vi "Teleop.vi"(10 "Match Info":T1={"Autonomous Elapsed Seconds"=0.0, "TeleOp Elapsed Seconds"=0.0, "Disabled Elapsed Seconds"=0.0, "Visited Autonomous"=FALSE, "Visited TeleOp"=FALSE, "Visited Disabled"=FALSE, "Autonomous Settings"={"Autonomous Style"=enum."Independent", "VI Refnum"=refnum}}, 11 "Call Context":T2) -> ()   [LabVIEW 2015]
doc: "This VI is called for each TeleOp packet received from the DS where the robot is not disabled. It is often used to read from the joysticks and update I/O or to update setpoints for timed control loops. It should complete and return within 20 milliseconds or it may miss DS packets."
uses:
  <vilib>/Rock Robotics/WPI/DriverStation/WPI_DriverStationDerivedRobotMode.ctl
  <vilib>/Rock Robotics/WPI/DriverStation/WPI_DriverStationMatch Info.ctl
  <vilib>/Rock Robotics/WPI/Utilities/WPI_GetSetVariantRefNum.vi
  <vilib>/Rock Robotics/Network Tables/SD Write Number.vi
  Robot Global Data.vi
  <vilib>/Rock Robotics/WPI/Solenoid/Deprecated/WPI_SolenoidSetBool.vi
  Z navX/navX Library v2/navX Library v2.lvlib
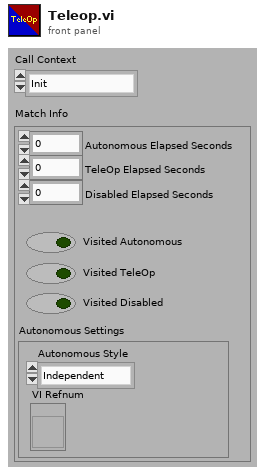
[diagram p1: front panel]
types:
  T1 = typedef "WPI_DriverStationMatch Info.ctl" = cluster{"Autonomous Elapsed Seconds":dbl, "TeleOp Elapsed Seconds":dbl, "Disabled Elapsed Seconds":dbl, "Visited Autonomous":bool, "Visited TeleOp":bool, "Visited Disabled":bool, "Autonomous Settings":cluster{"Autonomous Style":enum16{"Iterative", "Independent"}, "VI Refnum":refnum<vi>}}
  T2 = typedef "WPI_DriverStationDerivedRobotMode.ctl" = enum16{"Init", "Execute", "Stop"}
  T3 = enum16{"No Override", "Override to Coast", "Override to Brake"}
  T4 = typedef "WPI_JoystickDevRef.ctl" = cluster{"Device":T5}
  T5 = typedef "WPI_JoystickDeviceEnum.ctl" = enum16{"USB 0", "USB 1", "USB 2", "USB 3", "USB 4", "USB 5"}
  T6 = cluster{"Axes[0]":dbl, "Axes[1]":dbl, "Axes[2]":dbl, "Axes[3]":dbl, "Axes[4]":dbl, "Axes[5]":dbl, "Axes[6]":dbl, "Axes[7]":dbl, "Axes[8]":dbl}
  T7 = cluster{"Buttons[0]":bool, "Buttons[1]":bool, "Buttons[2]":bool, "Buttons[3]":bool, "Buttons[4]":bool, "Buttons[5]":bool, "Buttons[6]":bool, "Buttons[7]":bool, "Buttons[8]":bool}
  T8 = typedef "navX Library v2.lvlib/Z900_navX_DeviceTypeDef.ctl" = cluster{"Interface":cluster{"Protocol":T9, "Update Rate (4Hz-60Hz)":u8, "navX Open TypeDef":variant}, "Notify Packet":refnum<notifier>, "Loop VI Refnum":refnum<vi>, "Ready to Close Occurrence Refnum":refnum<k4>}
  T9 = typedef "navX Library v2.lvlib/Z900_navX_ProtocolTypeDef.ctl" = enum16{"SERIAL", "I2C", "SPI"}
  T10 = cluster{"Yaw":dbl, "Roll":dbl, "Pitch":dbl, "Heading":dbl, "Fused Heading":dbl}
  T11 = cluster{"LinearAcceleration X":dbl, "LinearAcceleration Y":dbl, "LinearAcceleration Z":dbl}
  T12 = cluster{"Velocity X":dbl, "Velocity Y":dbl, "Velocity Z":dbl, "Displacement X":dbl, "Displacement Y":dbl, "Displacement Z":dbl}
  T13 = typedef "WPI_MotorControlDeviceRef.ctl" = cluster{"DeviceStatus":errorcluster, "Type":T14, "PWM":cluster{"PWM Channel":T15, "DeadBand":T16}, "CAN":cluster{"Device Number":u8, "Control Mode":T17, "Semaphore":T18, "Max Vout":dbl, "TalonSRX Control Mode":T19}, "Invert":bool}
  T14 = typedef "WPI_MotorControlType.ctl" = enum16{"PWM", "CAN", "CANTalonSRX"}
  T15 = typedef "FPGA_DIOPWMChannel.ctl" = enum8{"PWM 0", "PWM 1", "PWM 2", "PWM 3", "PWM 4", "PWM 5", "PWM 6", "PWM 7", "PWM 8", "PWM 9", "PWM MXP 0", "PWM MXP 1", "PWM MXP 2", "PWM MXP 3", "PWM MXP 4", "PWM MXP 5", "PWM MXP 6", "PWM MXP 7", "PWM MXP 8", "PWM MXP 9", "Invalid"}
  T16 = typedef "WPI_PWMDeadband.ctl" = cluster{"Name":string, "maxPositivePwm":i32, "minPositivePwm":i32, "centerPwm":i32, "maxNegativePwm":i32, "minNegativePwm":i32, "angularRange":u16}
  T17 = typedef "WPI_CANJaguar_ControlMode.ctl" = enum8{"Percent VBus", "Current", "Speed", "Position", "Voltage"}
  T18 = typedef "Semaphore RefNum" = refnum<k1>
  T19 = typedef "WPI_CANTalonSRX_APIControlMode.ctl" = enum8{"Percent VBus", "Speed", "Position", "Slave", "Unchanged / Invalid", "Voltage Compensation", "Current", "Motion Profile"}
  T20 = typedef "WPI_SolenoidDevRef.ctl" = cluster{"DevStatus":errorcluster, "Pneumatics Control Module":u8, "Forward Solenoid Channel":T21, "Reverse Solenoid Channel":T21}
  T21 = typedef "WPI_SolenoidChannel.ctl" = enum8{"Solenoid 0", "Solenoid 1", "Solenoid 2", "Solenoid 3", "Solenoid 4", "Solenoid 5", "Solenoid 6", "Solenoid 7", "Invalid"}
  T22 = typedef "WPI_CANTalonSRX_GlobalStatus.ctl" = cluster{"Applied Throttle":dbl, "Module Enabled":bool, "CAN Error":errorcluster, "Closed Loop Error":dbl, "Forward Limit Switch Closed":bool, "Reverse Limit Switch Closed":bool, "Sensor Position":dbl, "Sensor Velocity":dbl, "Current":dbl, "Sticky Fault - Over Temp":bool, "Sticky Fault - Under Voltage":bool, "Sticky Fault - Forward Limit":bool, "Sticky Fault - Reverse Limit":bool, "Sticky Fault - Forward Soft Limit":bool, "Sticky Fault - Reverse Soft Limit":bool, "Brake is Enabled":bool, "Encoder Position":dbl, "Encoder Velocity":dbl, "Encoder Index Count":dbl, "Encoder A Pin State":bool, "Encoder B Pin State":bool, "Encoder Index Pin State":bool, "Analog In":dbl, "Analog In Velocity":dbl, "Temperature (C)":dbl, "Battery Voltage":dbl, "Control 5 Is Supported":bool, "Current Profile Slot Select":dbl, "Pos Div 8":bool, "Vel Div 4":bool, "Pulse Width Position":i32, "Pulse Width Velocity":i32, "Pulse Width Rise To Rise (us)":i32, "Pulse Width Rise To Fall (us)":i32, "Mot Prof Active Is Under Run":bool, "Mot Prof Active Has Under Run":bool, "Mot Prof Active Is Last":bool, "Mot Prof Active Velocity Only":bool, "Mot Prof Active Is Valid":bool, "Mot Prof Buffer Is Full":bool, "Mot Prof Active Profile Slot Select":i32, "Mot Prof NextID":i32, "Mot Prof Count":i32, "Mot Prof Active Velocity":dbl, "Mot Prof Active Position":dbl, "Mot Prof Output Enable":i32}
  T23 = typedef "WPI_RobotDriveDevRef.ctl" = cluster{"DevStatus":errorcluster, "Motors[]":T13[], "Square Inputs":bool, "Max Output":dbl}
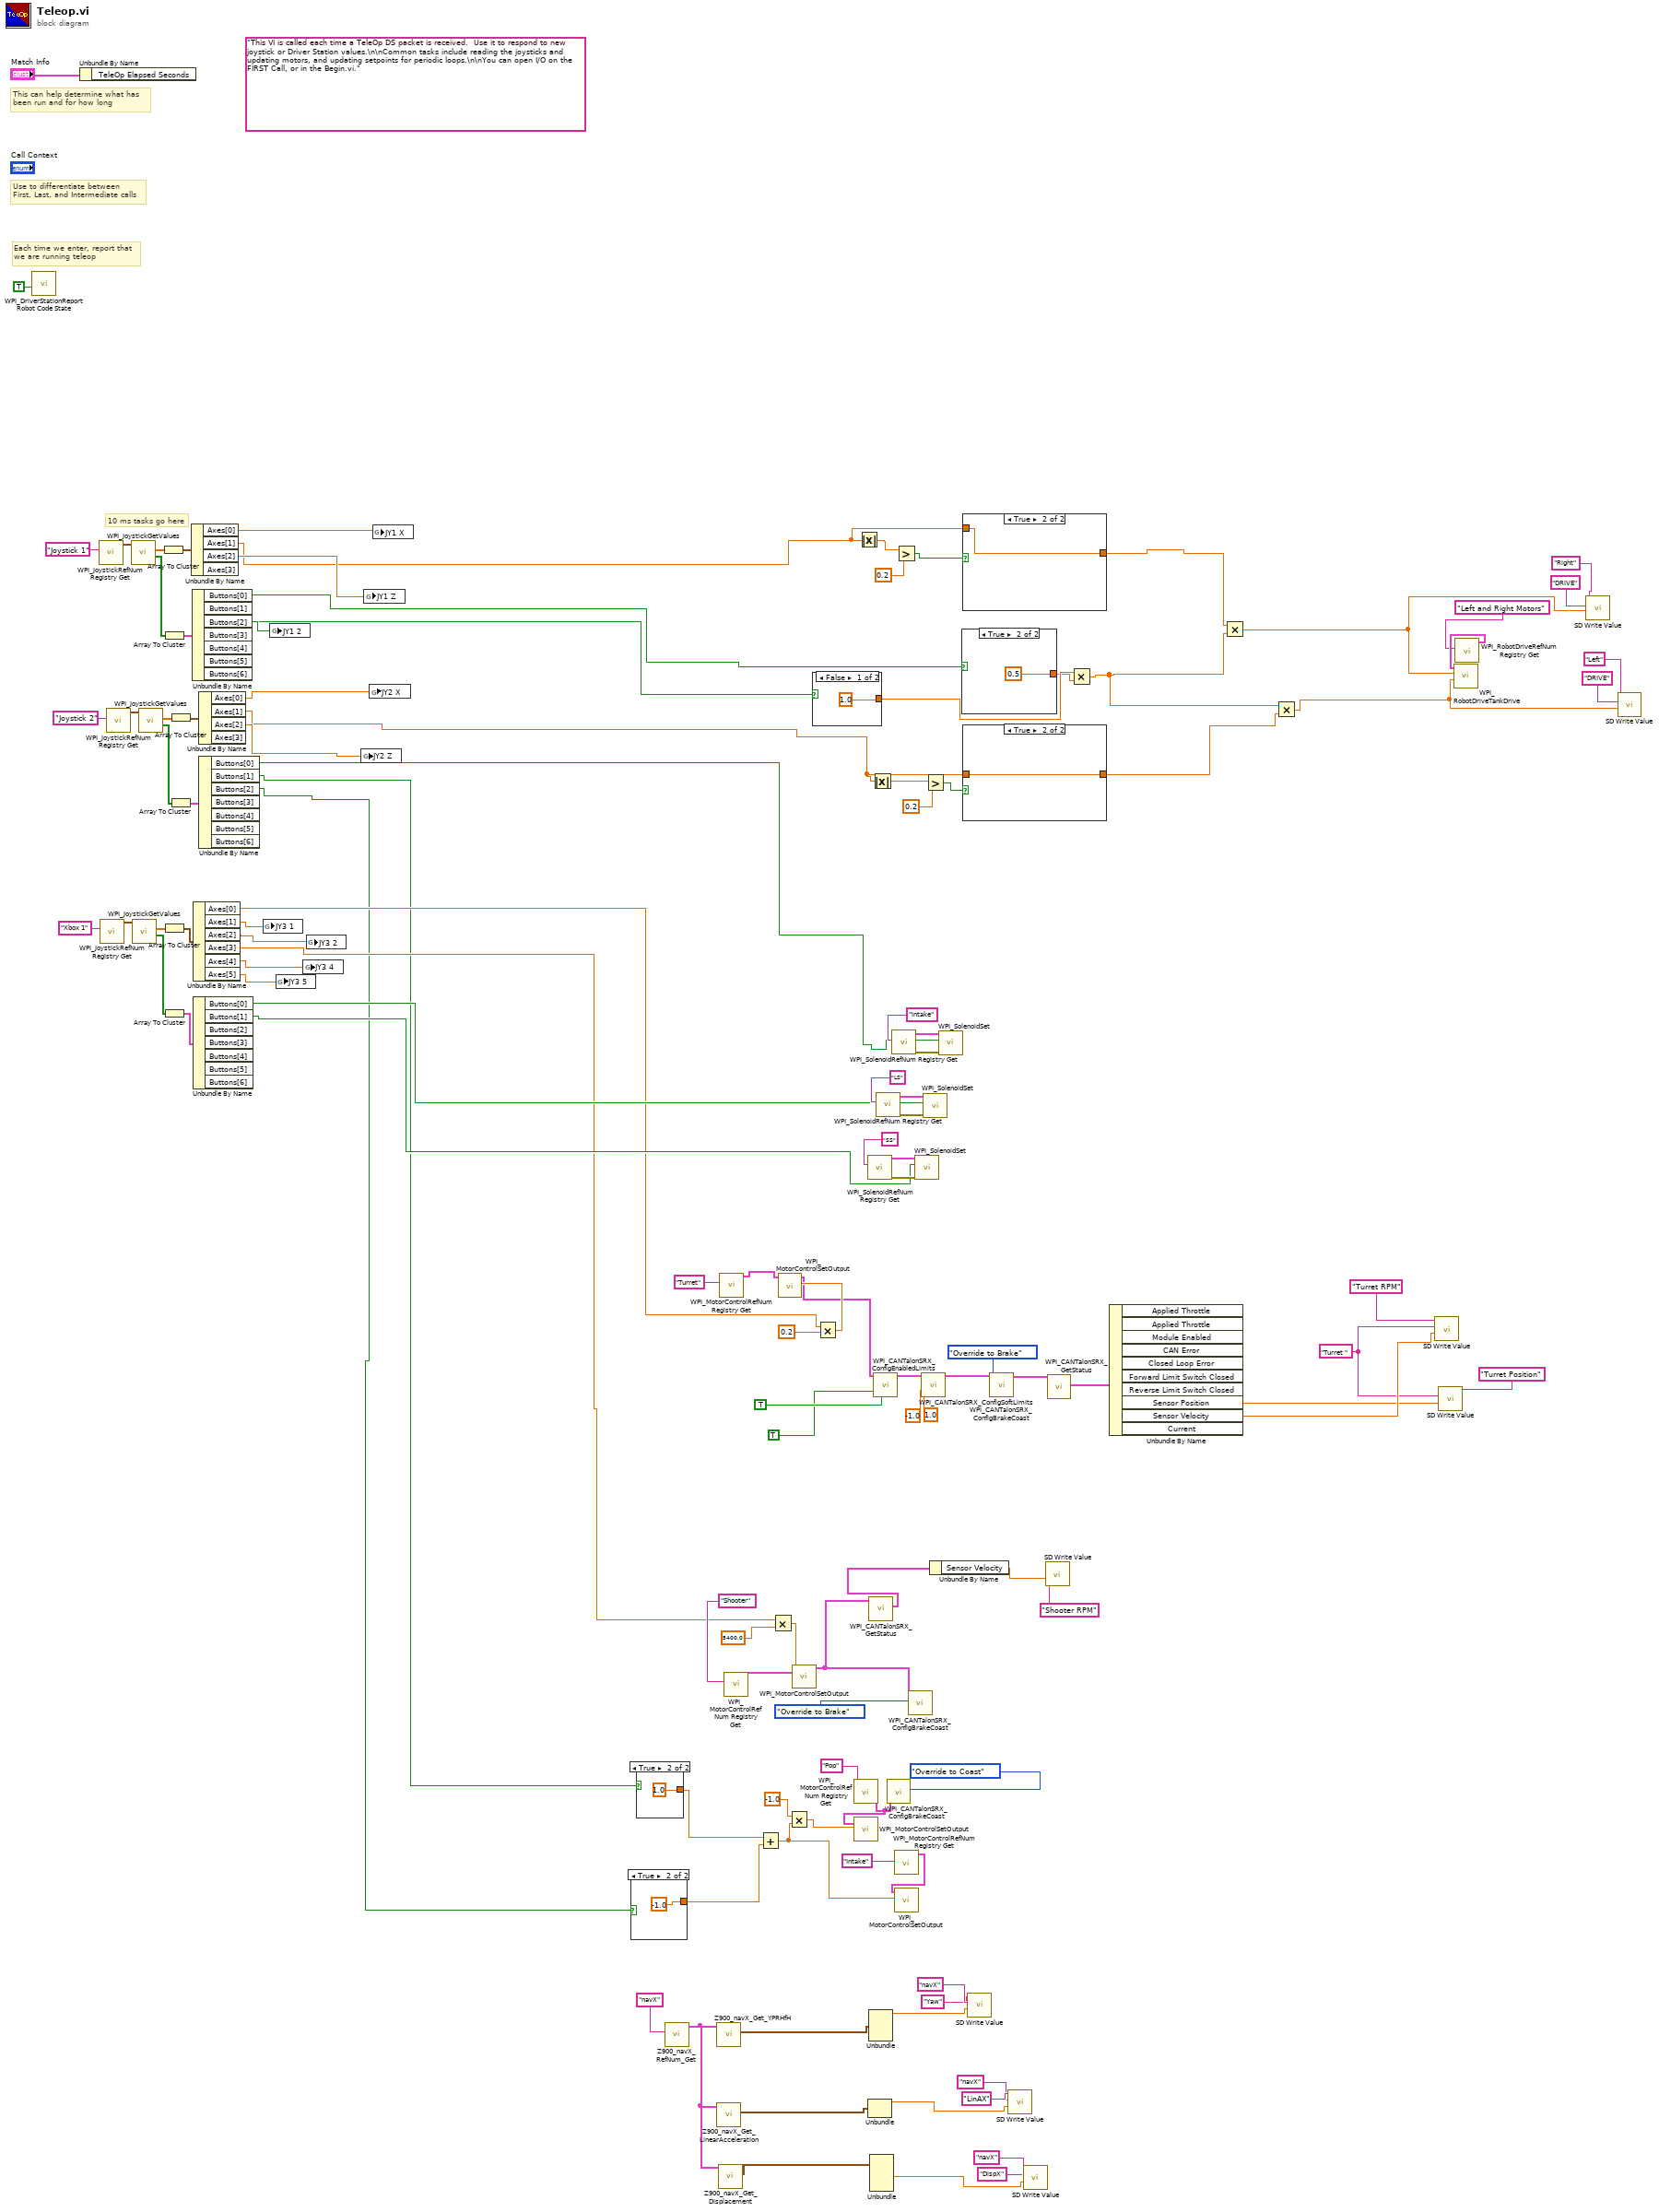
[diagram p0: block diagram]
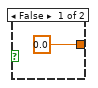
[diagram p2: hidden frame]
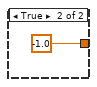
[diagram p3: hidden frame]
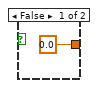
[diagram p4: hidden frame]
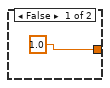
[diagram p5: hidden frame]
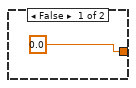
[diagram p6: hidden frame]
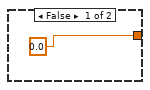
[diagram p7: hidden frame]
diagram:
  w9 = "Turret "
  (unwired) "This VI is called each time a TeleOp DS packet is received.  Use it to respond to new joystick or Driver Station values.\n\nCommon tasks include reading the joysticks and updating motors, and updating setpoints for periodic loops.\n\nYou can open I/O on the FIRST Call, or in the Begin.vi."
  # "10 ms tasks go here"
  # "Each time we enter, report that\nwe are running teleop"
  # "Use to differentiate between\nFirst, Last, and Intermediate calls"
  # "This can help determine what has\nbeen run and for how long"
  n1 = call <vilib>:"WPI_DriverStationReport Robot Code State.vi"("TeleOp"=TRUE ("Autonomous")) -> ()  [unwired: 10 in, 1 out]
  n2 = Unbundle By Name("Match Info") -> ()  [unwired: 1 out]
  n3 = call <vilib>:"WPI_JoystickRefNum Registry Get.vi"("refnum name"="Joystick 1") -> ("JoystickDevRef"=w70:T4)  [unwired: 1 in, 9 out]
  n4 = call <vilib>:"WPI_JoystickRefNum Registry Get.vi"("refnum name"="Xbox 1") -> ("JoystickDevRef"=w58:T4)  [unwired: 1 in, 9 out]
  n5 = call <vilib>:"WPI_JoystickRefNum Registry Get.vi"("refnum name"="Joystick 2") -> ("JoystickDevRef"=w64:T4)  [unwired: 1 in, 9 out]
  n6 = call <vilib>:"WPI_JoystickGetValues.vi"("JoystickDevRef"=w70) -> ("Buttons"=w68:bool[], "Axes"=w67:dbl[])  [unwired: 6 in, 3 out]
  n7 = call <vilib>:"WPI_JoystickGetValues.vi"("JoystickDevRef"=w58) -> ("Buttons"=w56:bool[], "Axes"=w55:dbl[])  [unwired: 6 in, 3 out]
  n8 = call <vilib>:"WPI_JoystickGetValues.vi"("JoystickDevRef"=w64) -> ("Buttons"=w62:bool[], "Axes"=w61:dbl[])  [unwired: 6 in, 3 out]
  n9 = Array To Cluster(array=w67) -> (cluster=w69:T6)
  n10 = Array To Cluster(array=w68) -> (cluster=w66:T7)
  n11 = Array To Cluster(array=w55) -> (cluster=w57:T6)
  n12 = Array To Cluster(array=w56) -> (cluster=w54:T7)
  n13 = Array To Cluster(array=w61) -> (cluster=w63:T6)
  n14 = Array To Cluster(array=w62) -> (cluster=w60:T7)
  n15 = Unbundle By Name(w69) -> ("Axes[0]"=w52:dbl, "Axes[1]"=w42:dbl, "Axes[2]"=w51:dbl)  [unwired: 1 out]
  n16 = Unbundle By Name(w66) -> ("Buttons[0]"=w44:bool, "Buttons[1]"=w43:bool, "Buttons[2]"=w45:bool)  [unwired: 4 out]
  n17 = Unbundle By Name(w57) -> ("Axes[0]"=w18:dbl, "Axes[1]"=w48:dbl, "Axes[2]"=w46:dbl, "Axes[3]"=w29:dbl, "Axes[4]"=w47:dbl, "Axes[5]"=w53:dbl)
  n18 = Unbundle By Name(w54) -> ("Buttons[0]"=w39:bool, "Buttons[1]"=w38:bool)  [unwired: 5 out]
  n19 = Unbundle By Name(w63) -> ("Axes[0]"=w50:dbl, "Axes[1]"=w41:dbl, "Axes[2]"=w49:dbl)  [unwired: 1 out]
  n20 = Unbundle By Name(w60) -> ("Buttons[0]"=w40:bool, "Buttons[1]"=w8:bool, "Buttons[2]"=w7:bool)  [unwired: 4 out]
  n21 = global write "Robot Global Data.vi" "JY3 1"(w48) -> ()
  n22 = global write "Robot Global Data.vi" "JY1 2"(w45) -> ()
  n23 = global write "Robot Global Data.vi" "JY3 5"(w53) -> ()
  n24 = global write "Robot Global Data.vi" "JY3 4"(w47) -> ()
  n25 = global write "Robot Global Data.vi" "JY3 2"(w46) -> ()
  n26 = global write "Robot Global Data.vi" "JY2 Z"(w49) -> ()
  n27 = global write "Robot Global Data.vi" "JY1 Z"(w51) -> ()
  n28 = global write "Robot Global Data.vi" "JY2 X"(w50) -> ()
  n29 = global write "Robot Global Data.vi" "JY1 X"(w52) -> ()
  n30 = case shown="True" w7 {
    tunnel: [0.0 -1.0] -> w85
    frame False {
    }
    frame True {
    }
  }
  n31 = case shown="True" w8 {
    tunnel: [0.0 1.0] -> w86
    frame False {
    }
    frame True {
    }
  }
  n32 = call "Z900_navX_RefNum_Get.vi"("refnum name"="navX") -> ("navX Device"=w35:T8)  [unwired: 9 in, 1 out]
  n33 = call "Z900_navX_Get_YPRHfH.vi"("navX Device"=w35) -> ("YRPHfH"=w36:T10)  [unwired: 7 in, 3 out]
  n34 = call "Z900_navX_Get_LinearAcceleration.vi"("navX Device"=w35) -> ("Linear Acceleration"=w34:T11)  [unwired: 7 in, 3 out]
  n35 = call "Z900_navX_Get_Displacement.vi"("navX Device"=w35) -> ("Displacement"=w33:T12)  [unwired: 7 in, 3 out]
  n36 = call <vilib>:"WPI_MotorControlRefNum Registry Get.vi"("refnum name"="Turret") -> ("MotorControlDevRef"=w17:T13)  [unwired: 9 in, 1 out]
  n37 = call <vilib>:"WPI_MotorControlRefNum Registry Get.vi"("refnum name"="Shooter") -> ("MotorControlDevRef"=w80:T13)  [unwired: 9 in, 1 out]
  n38 = Add(x=w86, y=w85) -> (x+y=w78:dbl)
  n39 = Multiply(x=w29, y=5400.0) -> (x*y=w84:dbl)
  n40 = Multiply(x=-1.0, y=w78) -> (x*y=w79:dbl)
  n41 = call <vilib>:"WPI_MotorControlSetOutput.vi"("Output"=w84, "MotorControlDevRef"=w80) -> ("MotorControlDevRef"=w75:T13)  [unwired: 7 in, 2 out]
  n42 = case shown="False" w43 {
    tunnel: [1.0 -1.0] -> w91
    frame False {
    }
    frame True {
    }
  }
  n43 = Multiply(x=w18, y=0.2) -> (x*y=w27:dbl)
  n44 = call <vilib>:"WPI_MotorControlSetOutput.vi"("Output"=w27, "MotorControlDevRef"=w17) -> ("MotorControlDevRef"=w16:T13)  [unwired: 7 in, 2 out]
  n45 = call <vilib>:"WPI_MotorControlRefNum Registry Get.vi"("refnum name"="Pop") -> ("MotorControlDevRef"=w73:T13)  [unwired: 9 in, 1 out]
  n46 = call <vilib>:"WPI_MotorControlSetOutput.vi"("Output"=w79, "MotorControlDevRef"=w73) -> ()  [unwired: 7 in, 3 out]
  n47 = Absolute Value(x=w42) -> (abs(x)=w114:dbl)
  n48 = call <vilib>:"WPI_SolenoidRefNum Registry Get.vi"("refnum name"="SS") -> ("error out"=w100:errorcluster, "SolenoidDevRef"=w101:T20)  [unwired: 9 in]
  n49 = Unbundle(w34) -> ("LinearAcceleration X"=w31:dbl)  [unwired: 2 out]
  n50 = call <vilib>:"WPI_CANTalonSRX_GetStatus.vi"("CAN Talon SRX Ref"=w75) -> ("Talon SRX Status"=w81:T22)  [unwired: 8 in, 2 out]
  n51 = Unbundle(w36) -> ("Yaw"=w32:dbl)  [unwired: 4 out]
  n52 = Unbundle(w33) -> ("Displacement X"=w30:dbl)  [unwired: 5 out]
  n53 = Absolute Value(x=w41) -> (abs(x)=w113:dbl)
  n54 = call <vilib>:"WPI_CANTalonSRX_ConfigEnabledLimits.vi"("CAN Talon SRX Ref"=w16, "Forward Soft Limit Enable"=TRUE, "Reverse Soft Limit Enable"=TRUE) -> ("CAN Talon SRX Ref"=w15:T13)  [unwired: 11 in, 1 out]
  n55 = call <vilib>:"WPI_SolenoidRefNum Registry Get.vi"("refnum name"="LS") -> ("error out"=w103:errorcluster, "SolenoidDevRef"=w104:T20)  [unwired: 9 in]
  n56 = call <vilib>:"WPI_CANTalonSRX_ConfigBrakeCoast.vi"("Brake / Coast Mode"=T3."Override to Coast", "CAN Talon SRX Ref"=w73) -> ()  [unwired: 8 in, 2 out]
  n57 = call <vilib>:"WPI_SolenoidRefNum Registry Get.vi"("refnum name"="Intake") -> ("error out"=w97:errorcluster, "SolenoidDevRef"=w98:T20)  [unwired: 9 in]
  n58 = Greater?(x=w114, y=0.2) -> (0:w118:bool)
  n59 = call <vilib>:"WPI_MotorControlRefNum Registry Get.vi"("refnum name"="Intake") -> ("MotorControlDevRef"=w87:T13)  [unwired: 9 in, 1 out]
  n60 = call <vilib>:"WPI_MotorControlSetOutput.vi"("Output"=w78, "MotorControlDevRef"=w87) -> ()  [unwired: 7 in, 3 out]
  n61 = call <vilib>:"WPI_CANTalonSRX_ConfigBrakeCoast.vi"("Brake / Coast Mode"=T3."Override to Brake", "CAN Talon SRX Ref"=w75) -> ()  [unwired: 8 in, 2 out]
  n62 = call-poly <vilib>:"WPI_SolenoidSet.vi"("error in (no error)"=w100, "Value"=w38, "SolenoidDevRef"=w101) -> ()  [unwired: 9 out]
  n63 = call <vilib>:"WPI_CANTalonSRX_ConfigSoftLimits.vi"("CAN Talon SRX Ref"=w15, "Forward Limit Position"=1.0, "Reverse Limit Position"=-1.0) -> ("CAN Talon SRX Ref"=w14:T13)  [unwired: 11 in, 1 out]
  n64 = call-poly <vilib>:"WPI_SolenoidSet.vi"("error in (no error)"=w103, "Value"=w39, "SolenoidDevRef"=w104) -> ()  [unwired: 9 out]
  n65 = Greater?(x=w113, y=0.2) -> (0:w116:bool)
  n66 = Unbundle By Name(w81) -> ("Sensor Velocity"=w82:dbl)
  n67 = call-poly <vilib>:"WPI_SolenoidSet.vi"("error in (no error)"=w97, "Value"=w40, "SolenoidDevRef"=w98) -> ()  [unwired: 9 out]
  n68 = case shown="True" w44 {
    tunnel: [1.0 0.5] -> w89
    frame False {
    }
    frame True {
    }
  }
  n69 = case shown="True" w118 {
    tunnel: [0.0 w130] -> w107
    tunnel: w42 -> [_ w130]
    frame False {
    }
    frame True {
    }
  }
  n70 = case shown="True" w116 {
    tunnel: [0.0 w132] -> w108
    tunnel: w41 -> [_ _]
    tunnel: w41 -> [_ w132]
    frame False {
    }
    frame True {
    }
  }
  n71 = call-poly <vilib>:"SD Write Value.vi"("Numeric"=w32, "Table Prefix"="navX", "Name"="Yaw") -> ()  [unwired: 7 in, 2 out]
  n72 = call <vilib>:"WPI_CANTalonSRX_ConfigBrakeCoast.vi"("Brake / Coast Mode"=T3."Override to Brake", "CAN Talon SRX Ref"=w14) -> ("CAN Talon SRX Ref"=w13:T13)  [unwired: 8 in, 1 out]
  n73 = call-poly <vilib>:"SD Write Value.vi"("Numeric"=w31, "Table Prefix"="navX", "Name"="LinAX") -> ()  [unwired: 7 in, 2 out]
  n74 = call-poly <vilib>:"SD Write Value.vi"("Numeric"=w30, "Table Prefix"="navX", "Name"="DispX") -> ()  [unwired: 7 in, 2 out]
  n75 = call-poly <vilib>:"SD Write Value.vi"("Numeric"=w82, "Table Prefix"="Shooter RPM") -> ()  [unwired: 8 in, 2 out]
  n76 = call <vilib>:"WPI_CANTalonSRX_GetStatus.vi"("CAN Talon SRX Ref"=w13) -> ("Talon SRX Status"=w12:T22)  [unwired: 8 in, 2 out]
  n77 = Multiply(x=w91, y=w89) -> (x*y=w90:dbl)
  n78 = Unbundle By Name(w12) -> ("Sensor Position"=w10:dbl, "Sensor Velocity"=w11:dbl)  [unwired: 8 out]
  n79 = Multiply(x=w107, y=w90) -> (x*y=w95:dbl)
  n80 = Multiply(x=w90, y=w108) -> (x*y=w94:dbl)
  n81 = call-poly <vilib>:"SD Write Value.vi"("Numeric"=w11, "Table Prefix"=w9, "Name"="Turret RPM") -> ()  [unwired: 7 in, 2 out]
  n82 = call-poly <vilib>:"SD Write Value.vi"("Numeric"=w10, "Table Prefix"=w9, "Name"="Turret Position") -> ()  [unwired: 7 in, 2 out]
  n83 = call <vilib>:"WPI_RobotDriveRefNum Registry Get.vi"("refnum name"="Left and Right Motors") -> ("RobotDriveDevRef"=w106:T23)  [unwired: 9 in, 1 out]
  n84 = call <vilib>:"WPI_RobotDriveTankDrive.vi"("Right axis value"=w94, "Left axis value"=w95, "RobotDriveDevRef"=w106) -> ()  [unwired: 6 in, 3 out]
  n85 = call-poly <vilib>:"SD Write Value.vi"("Numeric"=w95, "Table Prefix"="DRIVE", "Name"="Right") -> ()  [unwired: 7 in, 2 out]
  n86 = call-poly <vilib>:"SD Write Value.vi"("Numeric"=w94, "Table Prefix"="DRIVE", "Name"="Left") -> ()  [unwired: 7 in, 2 out]
